vi "_PC_Pub createFolder.vi"(8 "error in (no error)":errorcluster, 11 "path (use dialog)":path) -> (0 "error out":errorcluster, 3 "created path":path)   [LabVIEW 2018]
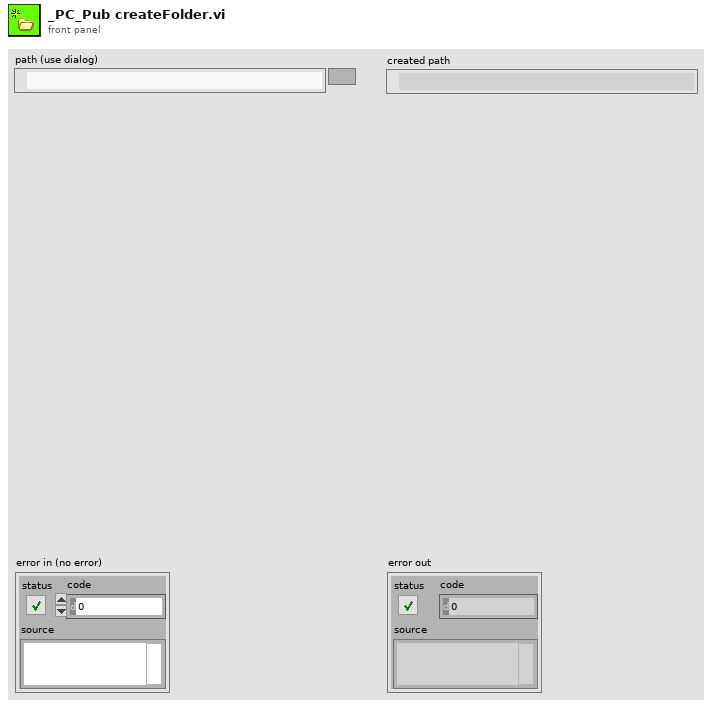
[diagram p1: front panel]
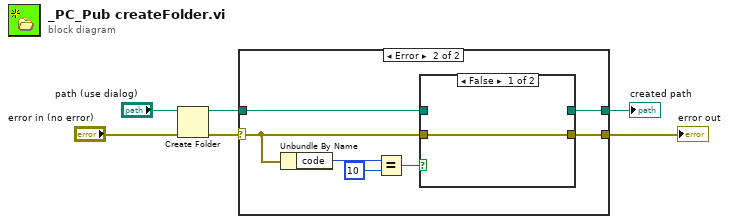
[diagram p0: block diagram]
diagram:
  n1 = Create Folder(path (use dialog)="path (use dialog)", error in="error in (no error)") -> (created path=w4:path, error out=w5:errorcluster)  [unwired: 1 in, 1 out]
  n2 = case shown="Error" w5 {
    selector: w5 -> [w7 w12]
    tunnel: w4 -> [w8 w11]
    tunnel: [w8 w10] -> w3
    tunnel: [w7 w9] -> w2
    frame No Error {
    }
    frame Error {
      n3 = Unbundle By Name(w12) -> ("code"=w15:i32)
      n4 = Equal?(x=w15, y=10) -> (x = y?=w13:bool)
      n5 = case shown="False" w13 {
        tunnel: w12 -> [w16 _]
        tunnel: w11 -> [_ w17]
        tunnel: [_ w17] -> w10
        tunnel: [w16 _] -> w9
        frame False {
        }
        frame True {
        }
      }
    }
  }
  "created path" <- w3
  "error out" <- w2
